vi "Node.Status.RT.Value.cpm.Movedone().vi"(11 ".NET Refnum in":refnum<k24>) -> ()   [LabVIEW 2020]
uses:
  C:/Users/Jonathan/Documents/Clearpath SDK/CSharp Examples/CLRWrapper/x64/Debug/CLRWrapper.dll
  CSharp Examples/CLRWrapper/x64/Debug/CLRWrapper.dll
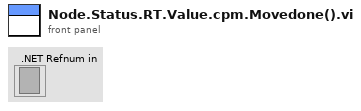
[diagram p1: front panel]
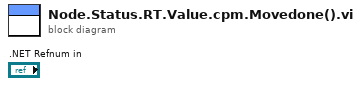
[diagram p0: block diagram]
diagram:
